vi "Message panel queue.vi"(2 "Action":enum16{"Initialise", "Add", "Read (& remove)"}(ring), 3 "New item":T1) -> (1 "Items removed from queue":T1[](array[typedef]))   [LabVIEW 2011]
uses:
  Message panel queue item.ctl
panel:
  out "Queue":T1[](array[typedef])
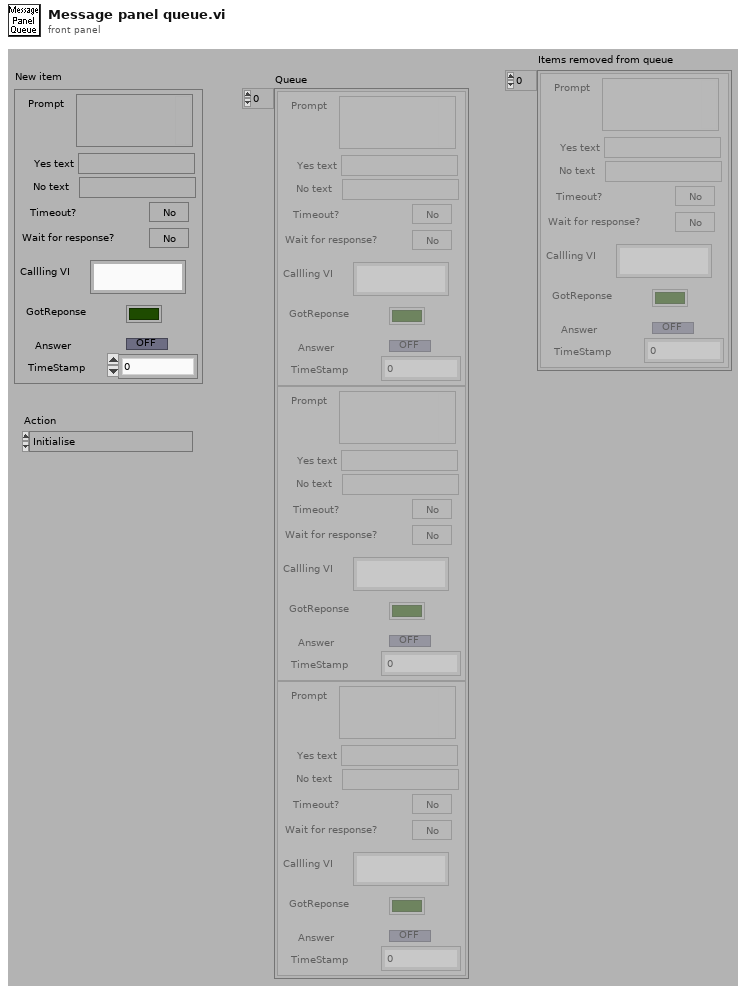
[diagram p1: front panel]
types:
  T1 = typedef "Message panel queue item.ctl" = cluster{"Prompt":string, "Yes text":string, "No text":string, "Timeout?":bool, "Wait for response?":bool, "Callling VI":string, "GotReponse":bool, "Answer":bool, "TimeStamp":u32}
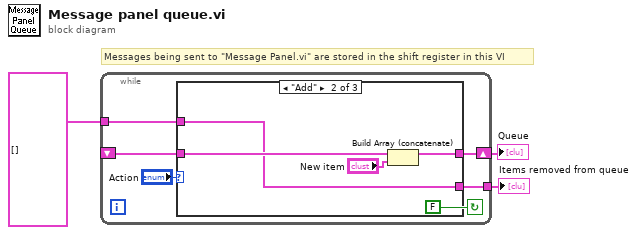
[diagram p0: block diagram]
diagram:
  # "Messages being sent to \"Message Panel.vi\" are stored in the shift register in this VI"
  n1 = while {
    shift-left: _ -> [w7]
    shift-right: [w8] -> w3
    tunnel: T1[] [] ("Queue in") -> [w5]
    tunnel: [w4] -> w1
    stop <- FALSE continue-if-true
    n2 = case shown="\"Add\"" "Action" {
      tunnel: [w10 w12 w16] -> w8
      tunnel: w7 -> [_ w14 w15]
      tunnel: w5 -> [w10 w11 w16]
      tunnel: [w10 w11 w15] -> w4
      frame "Initialise", Default {
      }
      frame "Add" {
        n3 = Build Array (concatenate)(w14, "New item") -> (w12:T1[])
      }
      frame "Read (& remove)" {
      }
    }
  }
  "Queue" <- w3
  "Items removed from queue" <- w1
